vi "Write Namer.vi"(8 "error in":errorcluster, 10 "Approval Tests.lvlib:Namer.lvclass":refnum<class "Namer.lvclass">, 11 "Options in":refnum<class "Options.lvclass">) -> (0 "error out":errorcluster, 3 "Options out":refnum<class "Options.lvclass">)   [LabVIEW 2020, in "Approval Tests.lvlib" / "Options.lvclass"]
uses:
  Options.lvclass
  Namer/Namer.lvclass
  Options.lvclass/Options.ctl
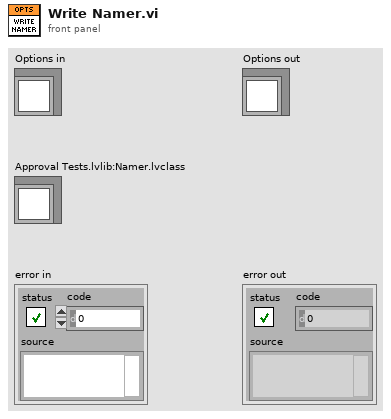
[diagram p1: front panel]
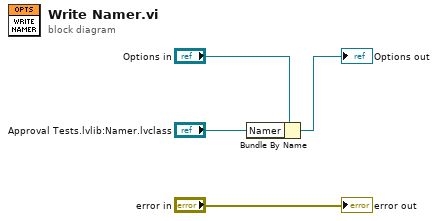
[diagram p0: block diagram]
diagram:
  n1 = Bundle By Name(cluster="Options in", "Namer"="Approval Tests.lvlib:Namer.lvclass") -> (→"Options out":refnum<class "Options.lvclass">)
  "error out" <- "error in"
